vi "Measure.vi"(5 "cancel refnum":refnum<vi>, 7 "error in (no error)":errorcluster, 8 "firmware revision":string(combo), 10 "VISA resource name":refnum<visa-resource-name>) -> (0 "error out":errorcluster, 1 "measurement results":T2, 2 "bridge error":T1, 3 "VISA resource name out":refnum<visa-resource-name>)   [LabVIEW 2024, in "Andeen-Hagerling 2700A.lvlib"]
doc: "Perform a single measurement and return the results in a cluster.\n\n<B>measurement results:</B>\n<B>error [I32]</B> - error code returned with the measurement (0 indincates no error).\n<B>frequency [DBL]</B> - frequency at which the measurement was performed.\n<B>capacitance [DBL]</B> - measured capacitance in units of pF.\n<B>loss [DBL]</B> - measured loss in the designated units. (refer to Set Units and Read Units VI's)\n<B>greater than [I32]</B> - In the case of parallel resistance (units GO) the greater than flag is used to indicate that the loss value represents the minimum resistance that the unknown impedance could have. Nonzero value indicates that greater than flag is set.\n<B>voltage [DBL]</B> - the voltage applied to the unknown during measurement."
uses:
  Andeen-Hagerling 2700A.lvlib
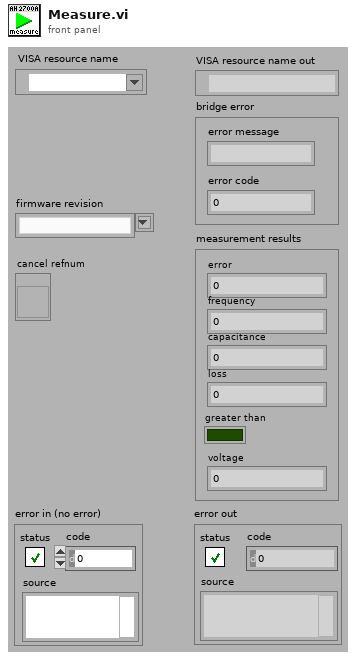
[diagram p1: front panel]
types:
  T1 = cluster{"error message":string, "error code":i32}
  T2 = cluster{"error":i32, "frequency":dbl, "capacitance":dbl, "loss":dbl, "greater than":bool, "voltage":dbl}
  T3 = cluster{"error code":i32, "frequency":dbl, "capacitance":dbl, "loss":dbl, "greater than":bool, "voltage":dbl}
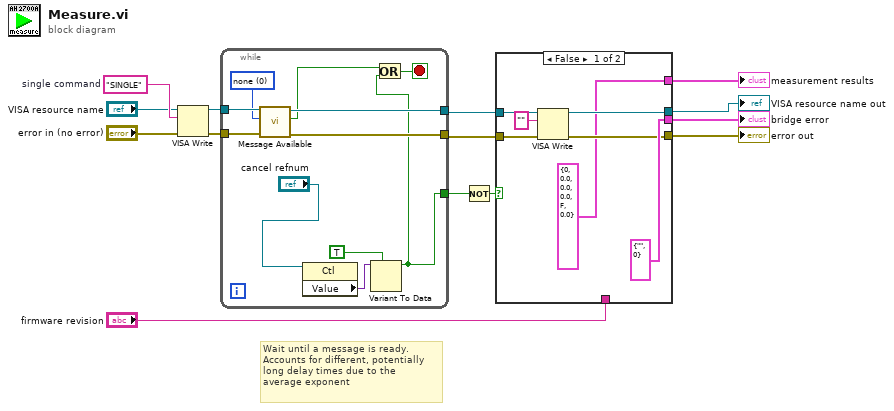
[diagram p0: block diagram]
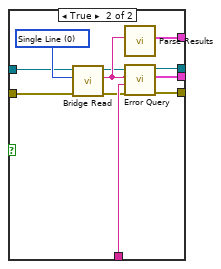
[diagram p2: hidden frame]
diagram:
  w14 = "SINGLE"  # single command
  # "Wait until a message is ready.\nAccounts for different, potentially\nlong delay times due to the \naverage exponent"
  n1 = VISA Write(VISA resource name="VISA resource name", write buffer=w14, error in (no error)="error in (no error)") -> (VISA resource name out=w6:refnum<visa-resource-name>, error out=w5:errorcluster)  [unwired: 1 out]
  n2 = while {
    tunnel: w6 -> [w25]
    tunnel: w5 -> [w24]
    tunnel: [w23] -> w4
    tunnel: [w22] -> w3
    tunnel: [w15] -> w1
    stop <- w20 stop-if-true
    w21 = u16 0 items=["none", "error check", "multiline read", "infinite"] ("delay")
    n3 = call "Message Available.vi"("error in (no error)"=w24, "delay"=w21, "VISA resource name"=w25) -> ("error out"=w22:errorcluster, "message available"=w19:bool, "VISA resource name out"=w23:refnum<visa-resource-name>)  [unwired: 6 in]
    n4 = property class="Ctl"(reference="cancel refnum") -> ("Value"=w17:variant)  [unwired: 1 in, 2 out]
    n5 = Variant To Data(type=TRUE, Variant=w17) -> (data=w15:bool)  [unwired: 1 in, 1 out]
    n6 = Or(x=w19, y=w15) -> (x .or. y?=w20:bool)
  }
  n7 = Not(x=w1) -> (.not. x?=w2:bool)
  n8 = case shown="False" w2 {
    tunnel: [T3 {"error code"=0, "frequency"=0.0, "capacitance"=0.0, "loss"=0.0, "greater than"=FALSE, "voltage"=0.0} ("measurement results") w43] -> w11
    tunnel: [w30 w42] -> w10
    tunnel: [w28 w41] -> w9
    tunnel: "firmware revision" -> [_ w40]
    tunnel: [T1 {"error message"="", "error code"=0} ("bridge error") w39] -> w7
    tunnel: w4 -> [w31 w34]
    tunnel: w3 -> [w29 w33]
    frame False {
      n9 = VISA Write(VISA resource name=w31, write buffer="", error in (no error)=w29) -> (VISA resource name out=w30:refnum<visa-resource-name>, error out=w28:errorcluster)  [unwired: 1 out]
    }
    frame True {
      w35 = u16 0 items=["Single Line", "Multi-Line"] ("Multiline")
      n10 = call "Bridge Read.vi"("error in (no error)"=w33, "multiline"=w35, "VISA resource name"=w34) -> ("error out"=w36:errorcluster, "read buffer"=w38:string, "VISA resource name out"=w37:refnum<visa-resource-name>)  [unwired: 6 in]
      n11 = call "Parse Results.vi"("measurement line"=w38) -> ("measurement results"=w43:T3)  [unwired: 9 in]
      n12 = call "Error Query.vi"("error in (no error)"=w36, "firmware revision"=w40, "measurement line"=w38, "VISA resource name"=w37) -> ("error out"=w41:errorcluster, "bridge error"=w39:T1, "VISA resource name out"=w42:refnum<visa-resource-name>)  [unwired: 5 in]
    }
  }
  "error out" <- w9
  "VISA resource name out" <- w10
  "measurement results" <- w11
  "bridge error" <- w7
